vi "Get SMO Name.vi"(8 "error in (no error)":errorcluster, 11 "instrument.PPMS3 in":refnum<class "instrument.PPMS3.lvclass">) -> (0 "error out":errorcluster, 2 "SMO Name":string, 3 "instrument.PPMS3 out":refnum<class "instrument.PPMS3.lvclass">)   [LabVIEW 2019, in "instrument.PPMS3.lvclass"]
uses:
  instrument.PPMS3.lvclass
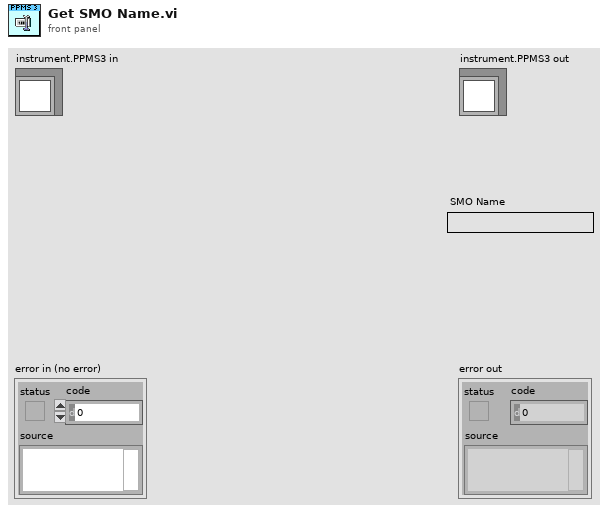
[diagram p1: front panel]
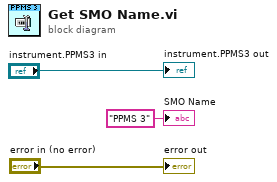
[diagram p0: block diagram]
diagram:
  "error out" <- "error in (no error)"
  "instrument.PPMS3 out" <- "instrument.PPMS3 in"
  "SMO Name" <- "PPMS 3" ("SMO Name")
